vi "Read Version.vi"(8 "error in (no error)":errorcluster, 11 "Measurement Client Wrapper in":refnum<class "Measurement Client Wrapper.lvclass">) -> (0 "error out":errorcluster, 2 "Version":string, 3 "Measurement Client Wrapper out":refnum<class "Measurement Client Wrapper.lvclass">)   [LabVIEW 2020, in "Measurement Client Wrapper.lvclass"]
uses:
  Measurement Client Wrapper.lvclass
  Measurement Client Wrapper.lvclass/Measurement Client Wrapper.ctl
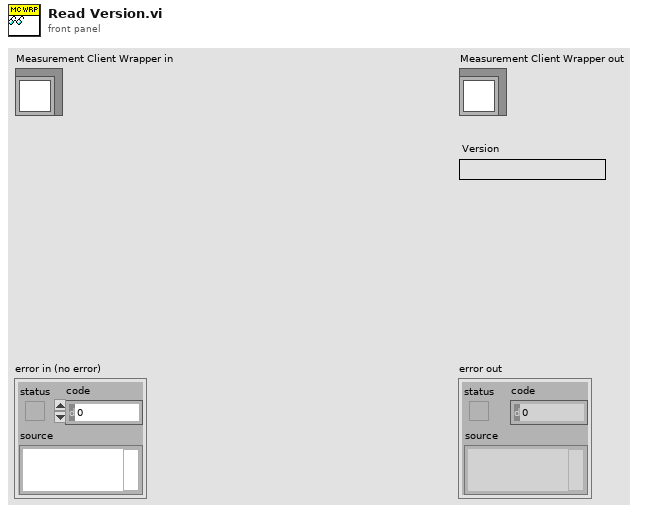
[diagram p1: front panel]
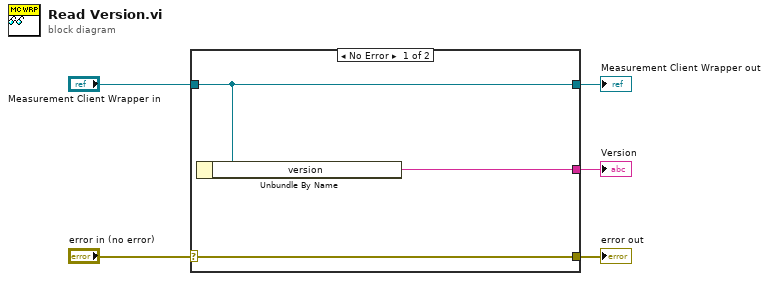
[diagram p0: block diagram]
diagram:
  n1 = case shown="No Error" "error in (no error)" {
    selector: "error in (no error)" -> [w8 w9]
    tunnel: [w8 w9] -> w4
    tunnel: [w7 w10] -> w2
    tunnel: "Measurement Client Wrapper in" -> [w7 w10]
    tunnel: [w6 _] -> w1
    frame No Error {
      n2 = Unbundle By Name(w7) -> ("version"=w6:string)
    }
    frame Error {
    }
  }
  "error out" <- w4
  "Measurement Client Wrapper out" <- w2
  "Version" <- w1
